vi "Slope Calibration Inputs.vi"(1 "Input":dbl format="%#_13g", 2 "Slope Calibration Inputs FGV Selector":T1, 3 "Action":T2) -> (0 "Output":dbl format="%#_13g")   [LabVIEW 2013]
uses:
  Action.ctl
  Slope Calibration Inputs FGV Selector.ctl
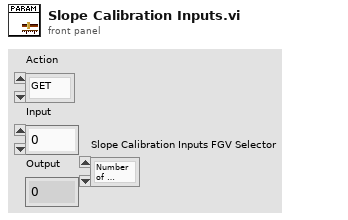
[diagram p1: front panel]
types:
  T1 = typedef "Slope Calibration Inputs FGV Selector.ctl" = enum16{"Number of Samples", "Ramp Rate", "Z Scan Size"}
  T2 = typedef "Action.ctl" = enum16{"GET", "PUT", "DELETE"}
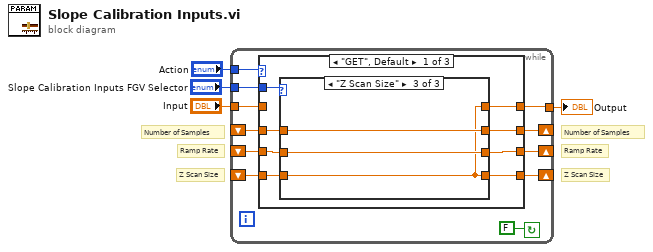
[diagram p0: block diagram]
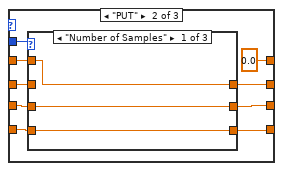
[diagram p4: hidden frame]
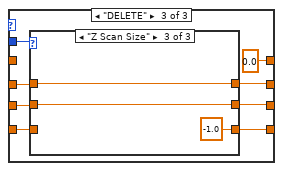
[diagram p7: hidden frame]
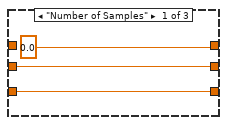
[diagram p8: hidden frame]
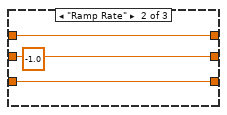
[diagram p9: hidden frame]
diagram:
  # "Z Scan Size"
  # "Z Scan Size"
  # "Ramp Rate"
  # "Number of Samples"
  # "Ramp Rate"
  # "Number of Samples"
  n1 = while {
    tunnel: "Action" -> [w14]
    tunnel: "Slope Calibration Inputs FGV Selector" -> [w13]
    shift-right: [w11] -> _
    shift-left: _ -> [w10]
    tunnel: "Input" -> [w7]
    tunnel: [w12] -> w2
    shift-right: [w9] -> _
    shift-left: _ -> [w8]
    shift-right: [w5] -> _
    shift-left: _ -> [w6]
    stop <- FALSE continue-if-true
    n2 = case shown="\"GET\", Default" w14 {
      tunnel: w13 -> [w23 w41 w53]
      tunnel: [w18 0.0 0.0] -> w12
      tunnel: [w22 w38 w56] -> w11
      tunnel: w10 -> [w21 w40 w58]
      tunnel: [w20 w37 w55] -> w9
      tunnel: w8 -> [w19 w39 w57]
      tunnel: w7 -> [_ w35 _]
      tunnel: [w17 w34 w52] -> w5
      tunnel: w6 -> [w16 w33 w51]
      frame "GET", Default {
        n3 = case shown="\"Z Scan Size\"" w23 {
          tunnel: [w25 w29 w32] -> w22
          tunnel: w21 -> [w25 w29 w32]
          tunnel: [w26 w28 w31] -> w20
          tunnel: w19 -> [w26 w28 w31]
          tunnel: [w25 w28 w30] -> w18
          tunnel: [w24 w27 w30] -> w17
          tunnel: w16 -> [w24 w27 w30]
          frame "Number of Samples" {
          }
          frame "Ramp Rate" {
          }
          frame "Z Scan Size" {
          }
        }
      }
      frame "PUT" {
        n4 = case shown="\"Number of Samples\"" w41 {
          tunnel: [w43 w47 w48] -> w38
          tunnel: w40 -> [_ w47 w48]
          tunnel: [w44 w46 w49] -> w37
          tunnel: w39 -> [w44 _ w49]
          tunnel: w35 -> [w43 w46 w50]
          tunnel: [w42 w45 w50] -> w34
          tunnel: w33 -> [w42 w45 _]
          frame "Number of Samples" {
          }
          frame "Ramp Rate" {
          }
          frame "Z Scan Size" {
          }
        }
      }
      frame "DELETE" {
        n5 = case shown="\"Z Scan Size\"" w53 {
          tunnel: [0.0 w64 w65] -> w56
          tunnel: w58 -> [_ w64 w65]
          tunnel: [w61 w63 w66] -> w55
          tunnel: w57 -> [w61 w63 w66]
          tunnel: [w59 w62 -1.0 ("Input")] -> w52
          tunnel: w51 -> [w59 w62 _]
          frame "Number of Samples" {
          }
          frame "Ramp Rate" {
            (unwired) -1.0
          }
          frame "Z Scan Size" {
          }
        }
      }
    }
  }
  "Output" <- w2
